vi "Modbus Gen.vi"(4 "Generator On":bool, 5 "Clear Alarms":bool, 6 "Error In 1":errorcluster, 7 "Error In 2":errorcluster) -> (0 "Error Out 1":errorcluster, 1 "Error Out 2":errorcluster, 2 "Gen Data Array":T1[](array[typedef]) {"Alarms" format="%04x"}, 3 "Gen Data":T1 {"Alarms" format="%04x"})   [LabVIEW 2014]
uses:
  Controls/Gen Data.ctl
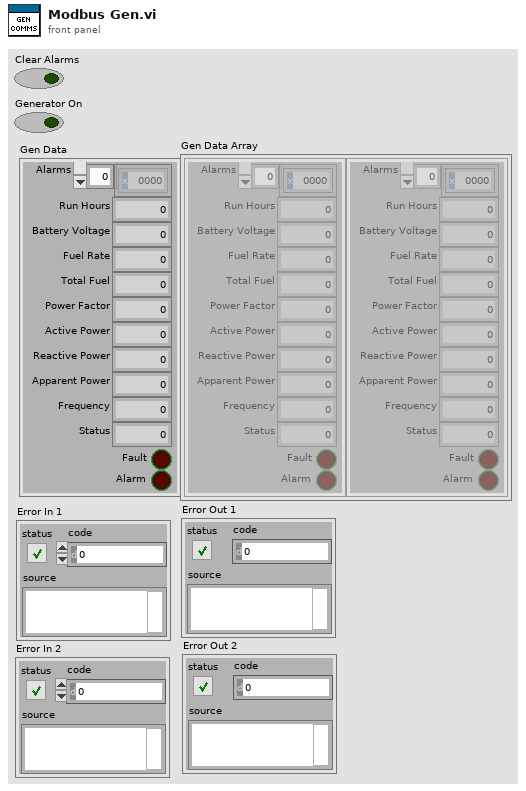
[diagram p1: front panel]
types:
  T1 = typedef "Gen Data.ctl" = cluster{"Alarms":i16[], "Run Hours":dbl, "Battery Voltage":dbl, "Fuel Rate":dbl, "Total Fuel":dbl, "Power Factor":dbl, "Active Power":dbl, "Reactive Power":dbl, "Apparent Power":dbl, "Frequency":dbl, "Status":i16, "Fault":bool, "Alarm":bool}
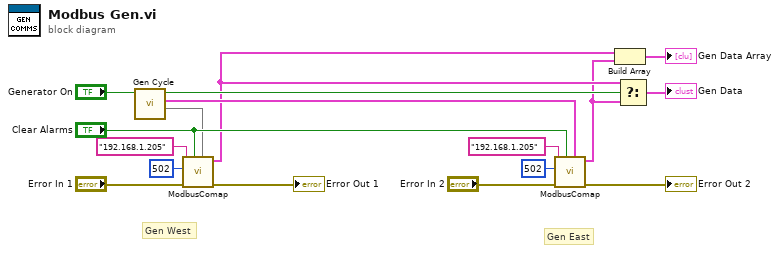
[diagram p0: block diagram]
diagram:
  # "Gen East"
  # "Gen West"
  n1 = call "Gen Cycle.vi"("Generator ON"="Generator On") -> (0:w9, "Gen Active"=w10:T1, "Generator ON West"=w11:bool)  [unwired: 7 in, 1 out]
  n2 = call <userlib>:"ModbusComap.vi"("Generator On"=w9, "Clear Alarms"="Clear Alarms", "Error In"="Error In 1", "port (502)"=u16 502, "address"="192.168.1.205") -> ("Error Out"=→"Error Out 1":errorcluster, "Gen Data"=w7:T1)  [unwired: 3 in]
  n3 = call <userlib>:"ModbusComap.vi"("Generator On"=w10, "Clear Alarms"="Clear Alarms", "Error In"="Error In 2", "port (502)"=u16 502, "address"="192.168.1.205") -> ("Error Out"=→"Error Out 2":errorcluster, "Gen Data"=w6:T1)  [unwired: 3 in]
  n4 = Build Array(w7, w6) -> (→"Gen Data Array":T1[])
  n5 = Select(t=w7, s=w11, f=w6) -> (s? t:f=→"Gen Data":T1)
